vi "DC Startup Settling Time Test.vi"(0 "TSM context":T1, 5 "Time to Capture (s)":dbl=0.015 format="%#_13g", 7 "Averaging Time (s)":dbl=0.002 format="%#_13g", 9 "Vdd Power On Voltage (V)":dbl=2.8 format="%#_13g", 11 "Vdd Current Range (A)":dbl=0.01 format="%#_13g", 12 "Debug Mode?":bool) -> (15 "error out":errorcluster)   [LabVIEW 2020]
doc: "VI determines the DC Startup settling time from Power ON till the required Vdc Level achieved on DUT output terminals."
uses:
  <vilib>/NI_TestStand_SemiconductorModule/NI_TestStand_Semiconductor_Module.lvlibp/PinMap/General/SemiconductorModuleContext.ctl
  <vilib>/NI_TestStand_SemiconductorModule/NI_TestStand_Semiconductor_Module.lvlibp/PinMap/TagProvider/TSM_Pin.ctl
  b970054a-d356-41b6-9493-53ae02ebcdc0.vi
  f04c93ba-d3a2-4f8d-88b4-688195d5f98d.vi
  5b21a69b-9d2c-48ab-967a-f84e1f0b8237.vi
  f7f5d33f-d09a-4d82-ae73-b91c36f905d8.vi
  f2bdec6b-afef-4d35-b3c0-e4111c9daaa3.vi
  b970054a-d356-41b6-9493-53ae02ebcdc0.vi/ae7c363b-d89c-43d0-be43-8f98b26b7c73.vi
  b970054a-d356-41b6-9493-53ae02ebcdc0.vi/6c82fdab-0884-43f6-8a73-47aee89b6396.vi
  b970054a-d356-41b6-9493-53ae02ebcdc0.vi/98738b93-12a5-4c37-98ad-0429d1868268.vi
  b970054a-d356-41b6-9493-53ae02ebcdc0.vi/947cc212-61f1-404f-b834-0b938824fb73.vi
  f04c93ba-d3a2-4f8d-88b4-688195d5f98d.vi/0594a305-9043-48cb-9582-0b21b588ec2f.vi
  f04c93ba-d3a2-4f8d-88b4-688195d5f98d.vi/57a46693-1186-41a2-8cec-46d83af6ce8c.vi
  f04c93ba-d3a2-4f8d-88b4-688195d5f98d.vi/d8299727-f7fc-485a-b5d1-a2a3829a9754.vi
  f04c93ba-d3a2-4f8d-88b4-688195d5f98d.vi/eed809dd-923b-4c52-8ded-6a5f52389026.vi
  Common/Instrument Control/DCPower/SSC DCPower/Source/Constant Voltage/SSC DCPower Force Voltage Array Symmetric Limits.vi
  <vilib>/measure/madcrms.llb/Basic Averaged DC-RMS for N Chan.vi
  <vilib>/NI_TestStand_SemiconductorModule/NI_TestStand_Semiconductor_Module.lvlibp/PinMap/General/Publish/PublishDataDoubleFunctionalTest.vi
  <vilib>/NI_TestStand_SemiconductorModule/NI_TestStand_Semiconductor_Module.lvlibp
  <vilib>/measure/NI_MAPro.lvlib
panel:
  out "DUT Out Voltage vs Time Graph":waveform(dbl)[](graph)
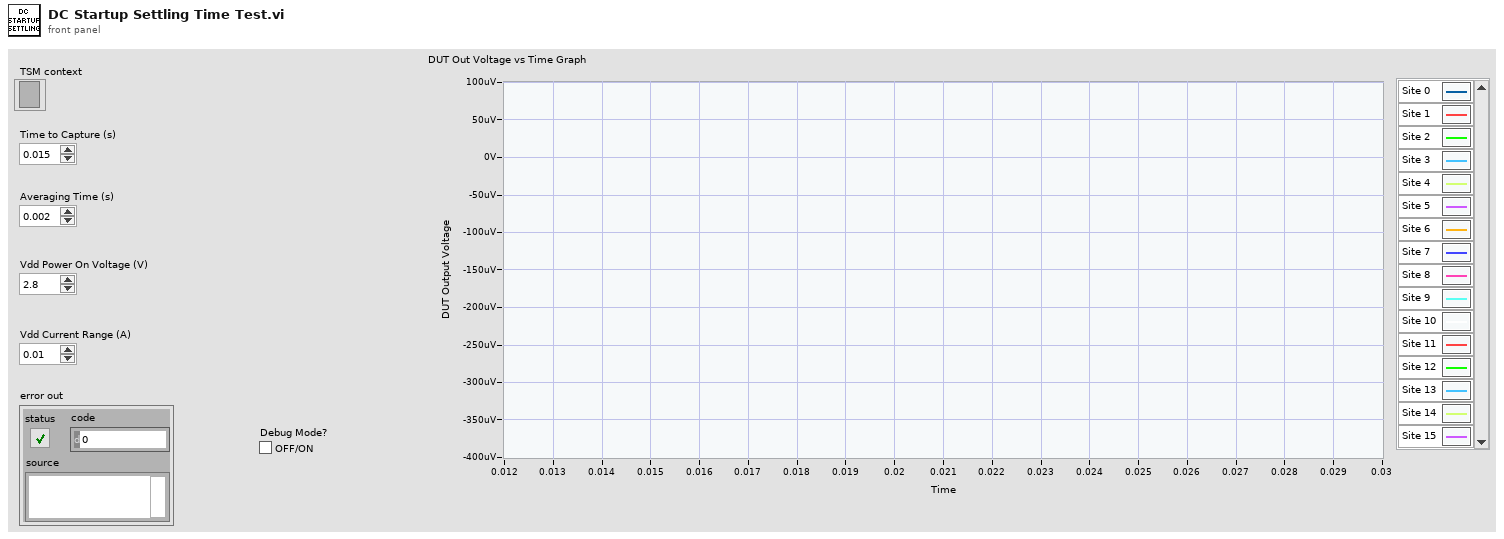
[diagram p1: front panel]
types:
  T1 = typedef "NI_TestStand_Semiconductor_Module.lvlibp/SemiconductorModuleContext.ctl" = refnum<k7>
  T2 = typedef "NI_TestStand_Semiconductor_Module.lvlibp/TSM_Pin.ctl" = tag
  T3 = typedef "TSM SSC DCPower.ctl" = cluster{"Pin Query Context":refnum<class "MultiplePinMultipleSessionQueryContext.lvclass">, "SSC":T4[], "Site Numbers":i32[], "Pins":T5[], "Pins Expanded":T7[]}
  T4 = typedef "SSC DCPower.ctl" = cluster{"Session":refnum<k15>, "Chan":string, "Channel List":string}
  T5 = typedef "TSM Pin Information.ctl" = cluster{"Pin":tag, "Type":T6, "Count":i32}
  T6 = typedef "TSM Pin Type Identifier.ctl" = enum8{"DUT Pin", "System Pin", "Pin Group", "Not Determined"}
  T7 = typedef "TSM Expanded Pin Information.ctl" = cluster{"Pin":tag, "Type":T6, "Index":i32}
  T8 = typedef "TSM DAQmx Multi-Task.ctl" = cluster{"Pin Query Context":refnum<class "MultiplePinMultipleSessionQueryContext.lvclass">, "SSC":T9[], "Site Numbers":i32[], "Pins":tag[]}
  T9 = typedef "SSC DAQmx.ctl" = cluster{"DAQmx Task ":refnum<k21>, "Channels":string, "Channel Lists":string}
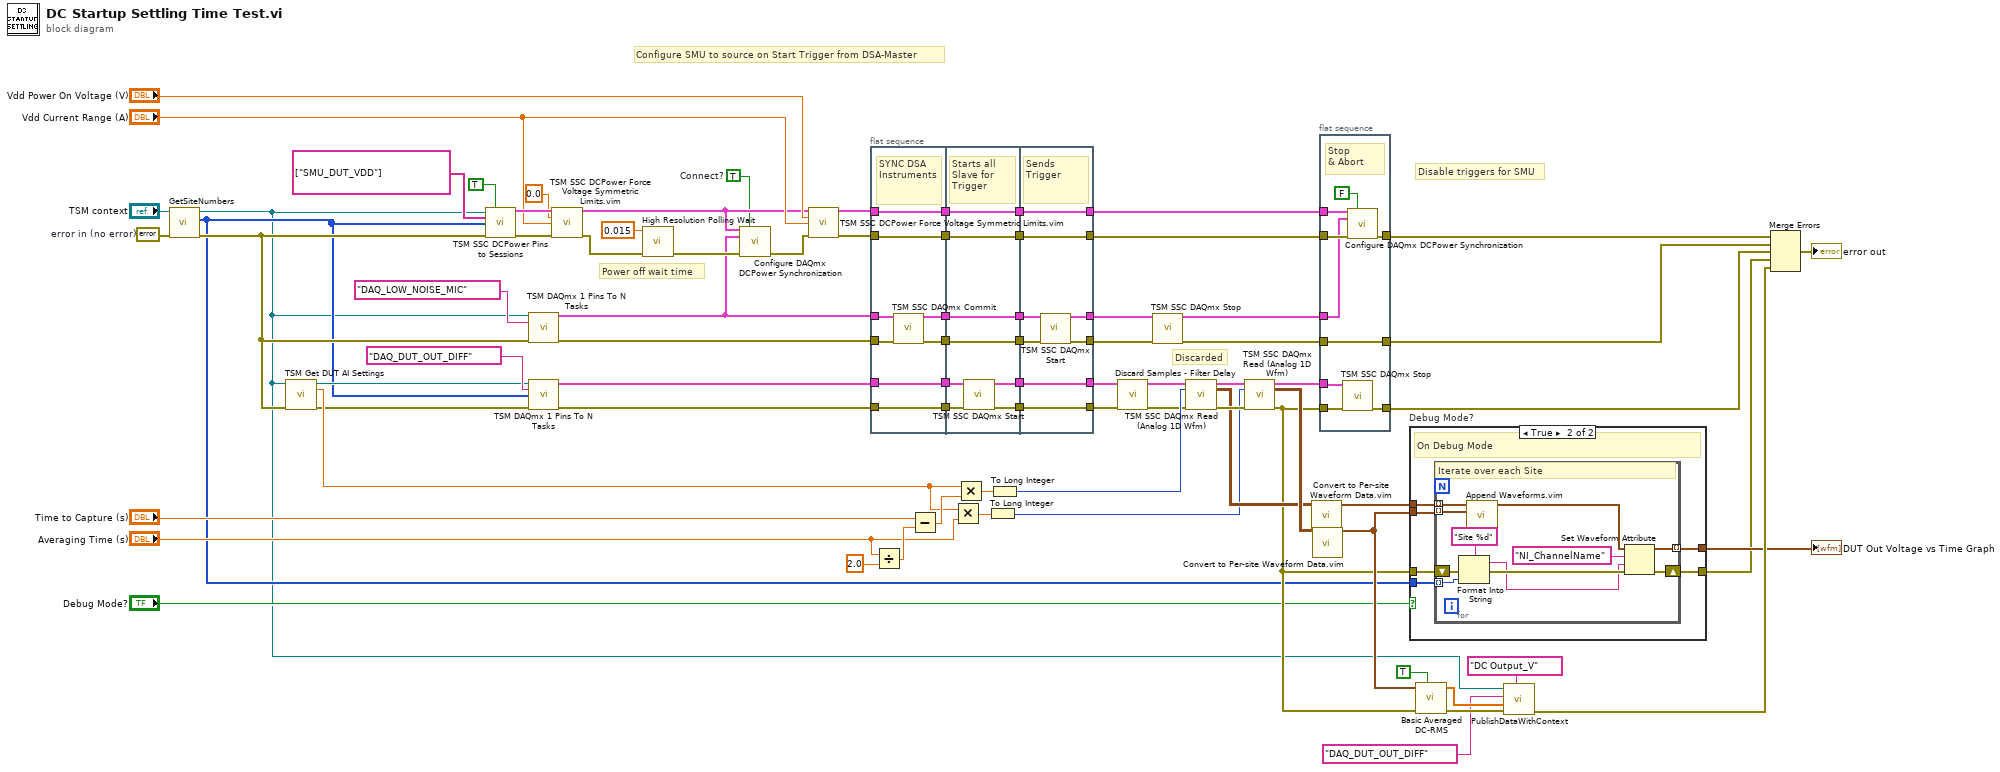
[diagram p0: block diagram]
diagram:
  w3 = TRUE  # Connect?
  w78 = errorcluster {"status"=FALSE, "code"=0, "source"=""}  # error in (no error)
  # "Configure SMU to source on Start Trigger from DSA-Master"
  # "Disable triggers for SMU"
  # "Discarded"
  # "Power off wait time"
  n1 = call <vilib>:"GetSiteNumbers.vi"("error in (no error)"=w78, "Semiconductor Module Context"="TSM context") -> ("error out"=w11:errorcluster, "Site Numbers"=w10:i32[], "Semiconductor Module Context Out"=w9:T1)  [unwired: 6 in, 1 out]
  n2 = call "TSM Get DUT AI Settings.vi"("TSM context"=w9, "error in (no error)"=w11) -> ("TSM context Out"=w28:T1, "Sampling Rate (Hz)"=w42:dbl, "error out"=w29:errorcluster)  [unwired: 9 in, 2 out]
  n3 = call "TSM SSC DCPower Pins to Sessions.vi"("TSM context"=w9, "Fill SSC Pin and Site Information? (T)"=TRUE, "Pins"=tag[] ["SMU_DUT_VDD"], "Site Numbers"=w10, "error in"=w11) -> ("DCPower TSM Out"=w55:T3, "error out"=w56:errorcluster)  [unwired: 9 in]
  n4 = call "TSM DAQmx 1 Pins To N Tasks.vi"("TSM context"=w9, "Pins"=tag "DAQ_LOW_NOISE_MIC", "error in"=w11) -> ("DAQ TSM Out"=w4:T8, "error out"=w62:errorcluster)  [unwired: 11 in]
  n5 = call "TSM DAQmx 1 Pins To N Tasks.vi"("TSM context"=w28, "Pins"=tag "DAQ_DUT_OUT_DIFF" ("DUT OUT Pin"), "Site Numbers"=w10, "error in"=w29) -> ("DAQ TSM Out"=w76:T8, "error out"=w75:errorcluster)  [unwired: 10 in]
  n6 = call "TSM SSC DCPower Force Voltage Symmetric Limits.vim"("DCPower TSM in"=w55, "Voltage Level (V)"=0.0, "Current Limit (A)"="Vdd Current Range (A)", "error in"=w56) -> ("DCPower TSM out"=w5:T3, "error out"=w54:errorcluster)  [unwired: 10 in]
  n7 = call <vilib>:"High Resolution Polling Wait.vi"("error in (no error)"=w54, "seconds to wait"=0.015) -> ("error out"=w52:errorcluster)  [unwired: 9 in]
  n8 = call "Configure DAQmx DCPower Synchronization.vi"("DCPower Trigger Destination"=w5, "Connect?"=w3, "DAQ Trigger Source"=w4, "error in (no error)"=w52) -> ("error out"=w6:errorcluster)  [unwired: 11 in]
  n9 = call "TSM SSC DCPower Force Voltage Symmetric Limits.vim"("DCPower TSM in"=w5, "Voltage Level (V)"="Vdd Power On Voltage (V)", "Current Limit (A)"="Vdd Current Range (A)", "error in"=w6) -> ("DCPower TSM out"=w51:T3, "error out"=w50:errorcluster)  [unwired: 10 in]
  n10 = flat-sequence {
    tunnel: w51 -> [w86]
    tunnel: w50 -> [w87]
    tunnel: w76 -> [w88]
    tunnel: w75 -> [w89]
    tunnel: [w89] -> w66
    tunnel: [w88] -> w65
    tunnel: [w87] -> w64
    tunnel: [w86] -> w63
    tunnel: w62 -> [w85]
    tunnel: w4 -> [w84]
    tunnel: [w83] -> w61
    tunnel: [w82] -> w60
    tunnel: [w91] -> w69
    tunnel: [w96] -> w68
    tunnel: [w94] -> w67
    tunnel: w66 -> [w97]
    tunnel: w65 -> [w95]
    tunnel: w64 -> [w91]
    tunnel: w63 -> [w90]
    tunnel: w61 -> [w92]
    tunnel: w60 -> [w93]
    tunnel: [w93] -> w59
    tunnel: [w92] -> w58
    tunnel: [w90] -> w49
    tunnel: [w104] -> w13
    tunnel: [w105] -> w40
    tunnel: [w99] -> w22
    tunnel: w69 -> [w99]
    tunnel: w68 -> [w105]
    tunnel: w67 -> [w104]
    tunnel: w59 -> [w103]
    tunnel: w58 -> [w102]
    tunnel: [w101] -> w27
    tunnel: [w100] -> w26
    tunnel: w49 -> [w98]
    tunnel: [w98] -> w2
    frame #0 {
      # "SYNC DSA Instruments"
      n11 = call "TSM SSC DAQmx Commit.vi"("TSM DAQmx In"=w84, "error in (no error)"=w85) -> ("TSM DAQmx Out"=w83:T8, "error out"=w82:errorcluster)  [unwired: 12 in]
    }
    frame #1 {
      # "Starts all Slave for Trigger"
      n12 = call "TSM SSC DAQmx Start.vi"("TSM DAQmx In"=w95, "error in (no error)"=w97) -> ("TSM DAQmx Out"=w94:T8, "error out"=w96:errorcluster)  [unwired: 12 in]
    }
    frame #2 {
      # "Sends Trigger"
      n13 = call "TSM SSC DAQmx Start.vi"("TSM DAQmx In"=w102, "error in (no error)"=w103) -> ("TSM DAQmx Out"=w100:T8, "error out"=w101:errorcluster)  [unwired: 12 in]
    }
  }
  n14 = Divide(x="Averaging Time (s)", y=2.0) -> (x/y=w45:dbl)
  n15 = Subtract(x="Time to Capture (s)", y=w45) -> (x-y=w44:dbl)
  n16 = Multiply(x=w42, y="Averaging Time (s)") -> (x*y=w41:dbl)
  n17 = Multiply(x=w42, y=w44) -> (x*y=w57:dbl)
  n18 = To Long Integer(number=w41) -> (32bit integer=w20:i32)
  n19 = To Long Integer(number=w57) -> (32bit integer=w21:i32)
  n20 = call "Discard Samples - Filter Delay.vi"("DAQ TSM in"=w13, "error in"=w40) -> ("DAQ TSM Out"=w12:T8, "error out"=w14:errorcluster)  [unwired: 12 in]
  n21 = call "TSM SSC DAQmx Stop.vi"("TSM DAQmx In"=w26, "error in (no error)"=w27) -> ("TSM DAQmx Out"=w1:T8, "error out"=w23:errorcluster)  [unwired: 12 in]
  n22 = call "TSM SSC DAQmx Read (Analog 1D Wfm).vi"("DAQ TSM in"=w12, "Samples to read"=w21, "error in"=w14) -> ("DAQ TSM Out"=w38:T8, "Per-Site Per-Pin Waveforms Out"=w37:waveform(dbl)[][], "error out"=w39:errorcluster)  [unwired: 10 in]
  n23 = call "TSM SSC DAQmx Read (Analog 1D Wfm).vi"("DAQ TSM in"=w38, "Samples to read"=w20, "error in"=w39) -> ("DAQ TSM Out"=w24:T8, "Per-Site Per-Pin Waveforms Out"=w80:waveform(dbl)[][], "error out"=w25:errorcluster)  [unwired: 10 in]
  n24 = call "Convert to Per-site Waveform Data.vim"("Per-Site Per-Pin Waveform In"=w37) -> ("Per-Site Waveform Out"=w33:waveform(dbl)[])  [unwired: 14 in]
  n25 = call "Convert to Per-site Waveform Data.vim"("Per-Site Per-Pin Waveform In"=w80) -> ("Per-Site Waveform Out"=w32:waveform(dbl)[])  [unwired: 14 in]
  n26 = flat-sequence {
    tunnel: w22 -> [w111]
    tunnel: [w110] -> _
    tunnel: w25 -> [w114]
    tunnel: [w113] -> w19
    tunnel: [w109] -> w17
    tunnel: w23 -> [w112]
    tunnel: [w112] -> w18
    tunnel: w24 -> [w110]
    tunnel: w2 -> [w108]
    tunnel: w1 -> [w106]
    frame #0 {
      # "Stop \n& Abort"
      n27 = call "TSM SSC DAQmx Stop.vi"("TSM DAQmx In"=w110, "error in (no error)"=w114) -> ("error out"=w113:errorcluster)  [unwired: 12 in, 1 out]
      n28 = call "Configure DAQmx DCPower Synchronization.vi"("DCPower Trigger Destination"=w108, "Connect?"=FALSE, "DAQ Trigger Source"=w106, "error in (no error)"=w111) -> ("error out"=w109:errorcluster)  [unwired: 11 in]
    }
  }
  n29 = case "Debug Mode?" shown="True" "Debug Mode?" {
    tunnel: w33 -> [_ w121]
    tunnel: w32 -> [_ w120]
    tunnel: [_ w119] -> w31
    tunnel: [w115 w118] -> w30
    tunnel: w25 -> [w115 w117]
    tunnel: w10 -> [_ w116]
    frame False {
      # "Normal Mode"
    }
    frame True {
      # "On Debug Mode"
      n30 = for {
        tunnel: w121 -> [w132] mode=indexing
        tunnel: w120 -> [w131] mode=indexing
        shift-right: [w124] -> w118
        shift-left: w117 -> [w126]
        tunnel: w116 -> [w123] mode=indexing
        tunnel: [w122] -> w119 mode=indexing
        # "Iterate over each Site"
        n31 = Format Into String(format string="Site %d", error in=w126, w123) -> (resulting string=w129:string, error out=w130:errorcluster)  [unwired: 1 in]
        n32 = call "Append Waveforms.vim"("Waveform A"=w132, "Waveform B"=w131) -> ("Appended Waveform Out"=w125:waveform(dbl))  [unwired: 13 in]
        n33 = Set Waveform Attribute(4:w130, 5:w129, 6:"NI_ChannelName" ("name"), 7:w125) -> (0:w124:errorcluster, 3:w122:waveform(dbl))  [unwired: 1 out]
      }
    }
  }
  "DUT Out Voltage vs Time Graph" <- w31
  n34 = call-poly <vilib>:"Basic Averaged DC-RMS.vi"("reset"=TRUE, "error in (no error)"=w25, "signals in"=w32) -> ("error out"=w35:errorcluster, "DC values"=w34:dbl[])  [unwired: 5 in, 2 out]
  n35 = call-poly <vilib>:"PublishDataWithContext.vi"("Published Data Id"=tag "DC Output_V", "error in (no error)"=w35, "Data In"=w34, "Pin"=T2 "DAQ_DUT_OUT_DIFF", "Semiconductor Module Context"=w9) -> ("error out"=w71:errorcluster)  [unwired: 5 in, 1 out]
  n36 = Merge Errors(w17, w18, w19, w30, w71) -> (→"error out":errorcluster)
